vi "Validate Instrument Revision.vi"(0 "VISA resource name":refnum<visa-resource-name>, 11 "error in (no error)":errorcluster) -> (4 "VISA resource name out":refnum<visa-resource-name>, 6 "Firmware Version":string, 10 "Ultra Models":enum16{"7800", "7804", "7820", "7850", "7854"}(ring), 15 "error out":errorcluster)   [LabVIEW 2020, in "Associated Research 78XX Series.lvlib"]
doc: "Queries the instrument for the model number and firmware revision and validates them."
uses:
  <instrlib>/Associated Research 78XX Series/Associated Research 78XX Series.lvlib
  <instrlib>/Associated Research 78XX Series/Private/ULTRA4 Model.ctl
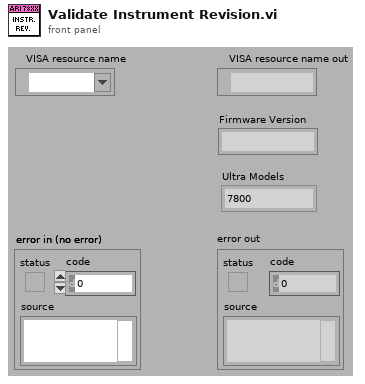
[diagram p1: front panel]
types:
  T1 = typedef "Associated Research 78XX Series.lvlib/ULTRA4 Model.ctl" = string[]
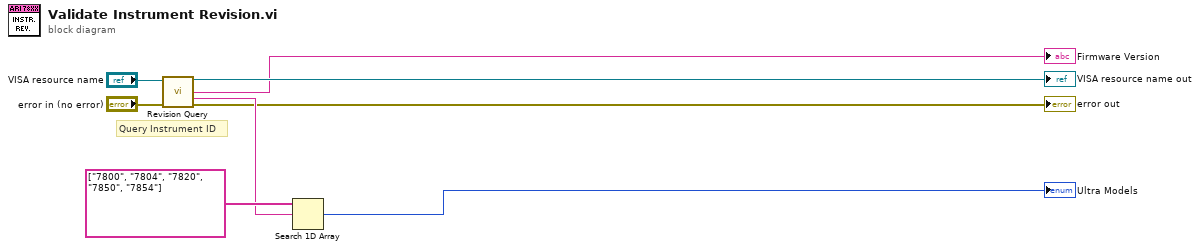
[diagram p0: block diagram]
diagram:
  # "Query Instrument ID"
  n1 = call <instrlib>:"Revision Query.vi"("VISA resource name"="VISA resource name", "error in (no error)"="error in (no error)") -> ("VISA resource name out"=→"VISA resource name out":refnum<visa-resource-name>, "Instrument Firmware Revision"=→"Firmware Version":string, "Instrument Model"=w5:string, "error out"=→"error out":errorcluster)  [unwired: 9 in, 1 out]
  n2 = Search 1D Array(1D array=T1 ["7800", "7804", "7820", "7850", "7854"] ("Instrument Models Supported"), element=w5) -> (index of element=→"Ultra Models":i32)  [unwired: 1 in]
